vi "As PropertyObject.vi"(8 "error in (no error)":errorcluster, 11 "PropertyObject in":refnum<class "PropertyObject.lvclass">) -> (0 "error out":errorcluster, 2 "PropertyObject":refnum<k7>, 3 "PropertyObject out":refnum<class "PropertyObject.lvclass">)   [LabVIEW 2020, in "TSnax.lvlib" / "PropertyObject.lvclass"]
uses:
  PropertyObject.lvclass
  PropertyObject.lvclass/PropertyObject.ctl
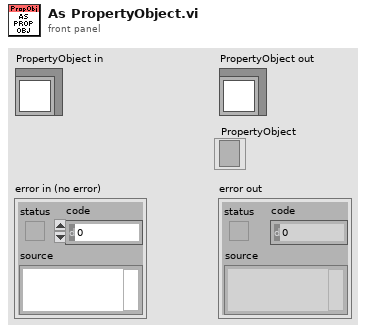
[diagram p1: front panel]
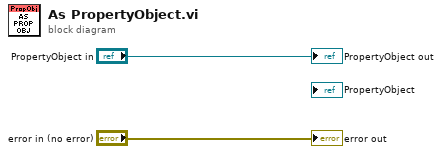
[diagram p0: block diagram]
diagram:
  "error out" <- "error in (no error)"
  "PropertyObject out" <- "PropertyObject in"
